vi "settings_to_ROI_info.vi"(8 "error in (no error)":errorcluster, 11 "TrajectoryMH100122AODRAPS in":refnum<class "TrajectoryMH100122AODRAPS.lvclass">) -> (0 "error out":errorcluster, 3 "TrajectoryMH100122AODRAPS out":refnum<class "TrajectoryMH100122AODRAPS.lvclass">)   [LabVIEW 2010, in "TrajectoryMH100122AODRAPS.lvclass"]
uses:
  TrajectoryMH100122AODRAPS.lvclass
  class_data.vi
  common/xcontrols/XImage/XImage/XImage.xctl
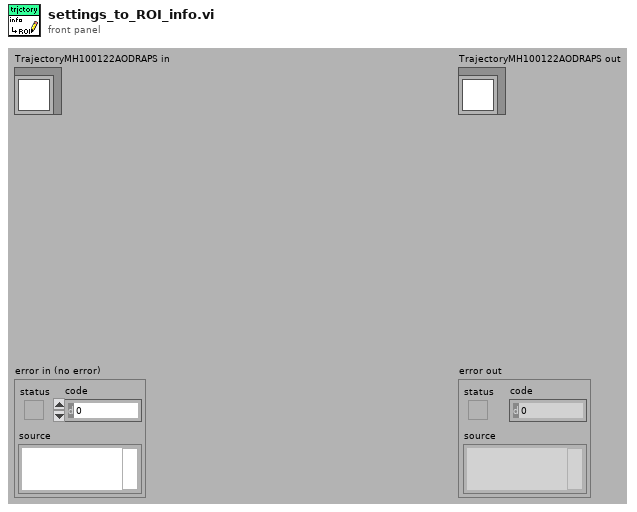
[diagram p1: front panel]
types:
  T1 = typedef "TrajectoryMH100122AODRAPS.lvclass/settings_cluster.ctl" = cluster{"no. of points":i32, "pixel dwell time":dbl[unit], "transformation factors":dbl[unit][], "2p imaging mirror switch":bool, "no. of frames":i32, "x resolution":u32, "zoom":dbl, "z angle (rotation angle, phi)":dbl[unit], "x angle (tilting angle, phi)":dbl[unit], "offset":dbl[unit][], "sub-pattern?":bool, "spiral radius":i8, "motion correction array size":u8, "y resolution":u32, "extrapolate line size":i32, "ROI color":u32, "line points color":u32, "z-step size / frame":u16, "z-offset":u16, "ROI numbering":bool, "winding number":dbl, "number of iteration points":dbl, "height":dbl, "amp":dbl}
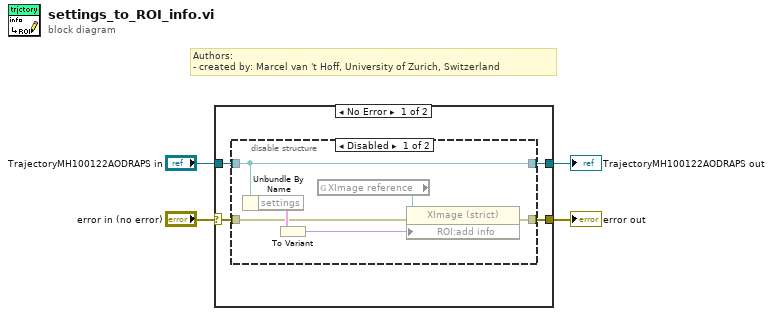
[diagram p0: block diagram]
diagram:
  # "Authors: \n- created by: Marcel van 't Hoff, University of Zurich, Switzerland"
  n1 = case shown="No Error" "error in (no error)" {
    selector: "error in (no error)" -> [w7 w18]
    tunnel: [w6 w18] -> w3
    tunnel: [w5 w17] -> w1
    tunnel: "TrajectoryMH100122AODRAPS in" -> [w8 w17]
    frame No Error {
      n2 = disable-structure shown="Disabled" {
        disable-tunnel: w8 -> [w9 w16]
        disable-tunnel: w7 -> [w11 w15]
        disable-tunnel: [w10 w15] -> w6
        disable-tunnel: [w9 w16] -> w5
        frame Disabled {
          n3 = Unbundle By Name(w9) -> ("settings"=w12:T1)
          n4 = To Variant(anything=w12) -> (Variant=w13:variant)
          n5 = global read "class_data.vi" "XImage reference"() -> (w14:refnum<vi>)
          n6 = property class="XImage (strict)"(reference=w14, error in=w11, "ROI:add info"=w13) -> (error out=w10:errorcluster)  [unwired: 1 out]
        }
        frame Enabled {
        }
      }
    }
    frame Error {
    }
  }
  "error out" <- w3
  "TrajectoryMH100122AODRAPS out" <- w1
